vi "Stop Looping.vi"(8 "error in (no error)":errorcluster, 11 "Helper Loop in":refnum<class "Helper Loop.lvclass">) -> (0 "error out":errorcluster, 3 "Helper Loop out":refnum<class "Helper Loop.lvclass">)   [LabVIEW 2024, in "Helper Loop.lvlib" / "Helper Loop.lvclass"]
uses:
  Helper Loop.lvclass
  Helper Loop.lvclass/Helper Loop.ctl
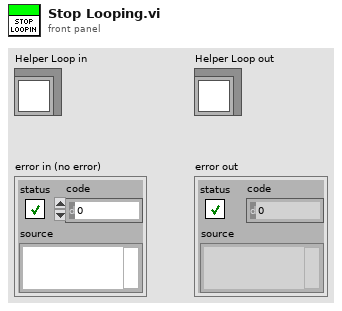
[diagram p1: front panel]
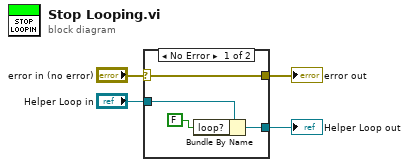
[diagram p0: block diagram]
diagram:
  n1 = case shown="No Error" "error in (no error)" {
    selector: "error in (no error)" -> [w8 w10]
    tunnel: [w8 w10] -> w3
    tunnel: [w5 w9] -> w1
    tunnel: "Helper Loop in" -> [w7 w9]
    frame No Error {
      n2 = Bundle By Name(cluster=w7, "loop?"=FALSE) -> (w5:refnum<class "Helper Loop.lvclass">)
    }
    frame Error {
    }
  }
  "error out" <- w3
  "Helper Loop out" <- w1
